vi "Parse file name.vi"(10 "filename without extension":string, 11 "File Path":path) -> (1 "Changed reg":u8, 2 "Part info":string[](array[string]), 3 "Part info Header":string[](array[string]))   [LabVIEW 2020]
uses:
  XML Handler/XML Handler.lvclass
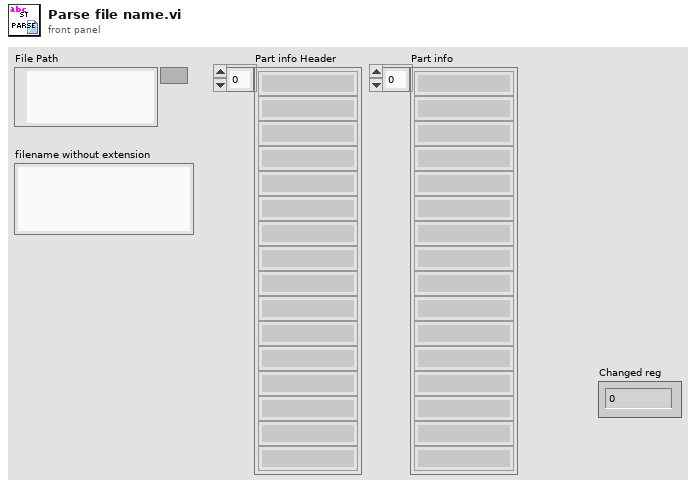
[diagram p1: front panel]
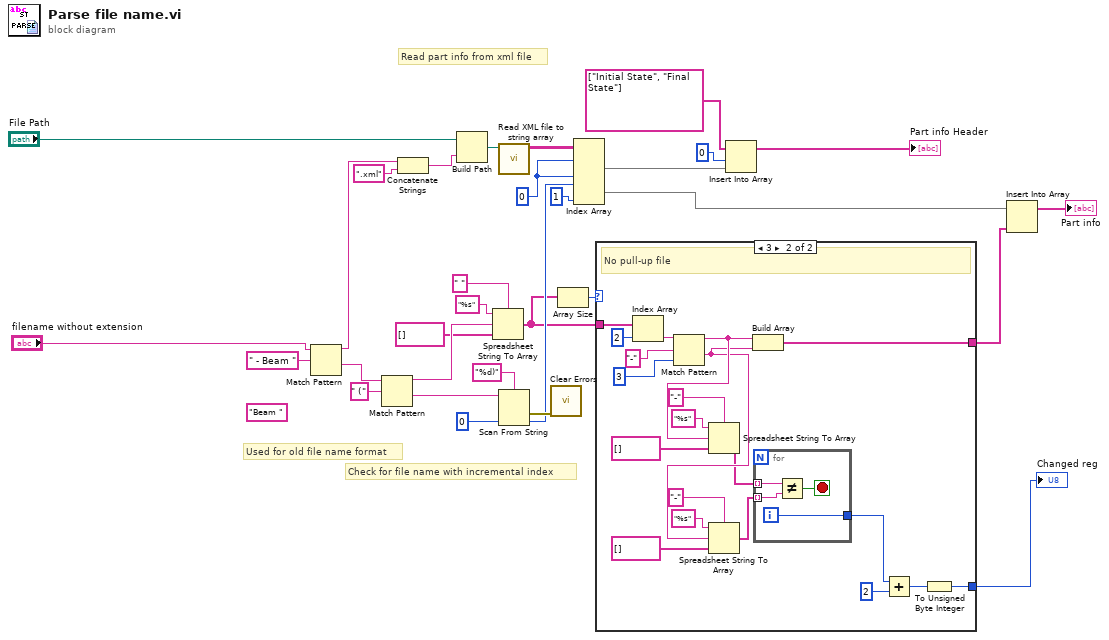
[diagram p0: block diagram]
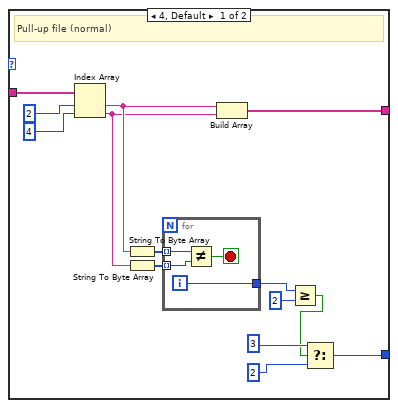
[diagram p2: hidden frame]
diagram:
  (unwired) "Beam " ("regular expression")
  w23 = 0 ("disabled index (page)")
  # "Used for old file name format"
  # "Check for file name with incremental index"
  # "Read part info from xml file"
  n1 = Match Pattern(string="filename without extension", regular expression=" - Beam ") -> (before substring=w25:string, after substring=w30:string)  [unwired: 1 in, 2 out]
  n2 = Match Pattern(string=w30, regular expression=" (") -> (before substring=w19:string, after substring=w18:string)  [unwired: 1 in, 2 out]
  n3 = Concatenate Strings(w25, ".xml" ("string")) -> (w24:string)
  n4 = Build Path(base path="File Path", name or relative path=w24) -> (appended path=w31:path)
  n5 = Spreadsheet String To Array(delimiter (Tab)=" ", format string="%s", spreadsheet string=w19, array type (2D Dbl)=string[] []) -> (array=w6:string[])
  n6 = call "Read XML file to string array.vi"("path to XML document"=w31) -> ("Array"=w11:string[][][])  [unwired: 9 in, 1 out]
  n7 = Scan From String(format string="%d)", input string=w18, default 1=0 ("default value 1")) -> (error out=w22:errorcluster, output 1=w21:i32)  [unwired: 2 in, 2 out]
  n8 = call <vilib>:"Clear Errors.vi"("error in (no error)"=w22) -> ()  [unwired: 5 in, 2 out]
  n9 = Array Size(array=w6) -> (size(s)=w5:i32)
  n10 = Index Array(array=w11, index (dim 0) #1=w23, index (dim 2) #1=w23, index (dim 0) #2=w21, index (dim 2) #2=1 ("disabled index (col)")) -> (element #1=w9:string[], element #2=w3:string[])  [unwired: 2 in]
  n11 = case shown="3" w5 {
    tunnel: w6 -> [w45 w69]
    tunnel: [w42 w64] -> w4
    tunnel: [w34 w50] -> w1
    frame 4, Default {
      # "Pull-up file (normal)"
      n12 = Index Array(array=w45, index #1=2 ("index"), index #2=4 ("index")) -> (element #1=w33:string, element #2=w32:string)
      n13 = String To Byte Array(string=w33) -> (unsigned byte array=w41:u8[])
      n14 = String To Byte Array(string=w32) -> (unsigned byte array=w40:u8[])
      n15 = for {
        tunnel: w41 -> [w49] mode=indexing
        tunnel: w40 -> [w48] mode=indexing
        tunnel: [w46] -> w39
        i -> [w46]
        stop <- w47 stop-if-true
        n16 = Not Equal?(x=w49, y=w48) -> (x != y?=w47:bool)
      }
      n17 = Build Array(w33, w32) -> (w42:string[])
      n18 = Greater Or Equal?(x=w39, y=2) -> (x >= y?=w35:bool)
      n19 = Select(t=u8 3, s=w35, f=u8 2) -> (s? t:f=w34:u8)
    }
    frame 3 {
      # "No pull-up file"
      n20 = Index Array(array=w69, index=2) -> (element=w67:string)
      n21 = Match Pattern(string=w67, regular expression="-", offset (0)=3) -> (before substring=w57:string, after substring=w56:string)  [unwired: 2 out]
      n22 = Spreadsheet String To Array(delimiter (Tab)="-", format string="%s", spreadsheet string=w57, array type (2D Dbl)=string[] []) -> (array=w54:string[])
      n23 = Spreadsheet String To Array(delimiter (Tab)="-", format string="%s", spreadsheet string=w56, array type (2D Dbl)=string[] []) -> (array=w55:string[])
      n24 = Build Array(w57, w56) -> (w64:string[])
      n25 = for {
        tunnel: w54 -> [w73] mode=indexing
        tunnel: w55 -> [w72] mode=indexing
        tunnel: [w70] -> w53
        i -> [w70]
        stop <- w71 stop-if-true
        n26 = Not Equal?(x=w73, y=w72) -> (x != y?=w71:bool)
      }
      n27 = Add(x=w53, y=2) -> (x+y=w51:i32)
      n28 = To Unsigned Byte Integer(number=w51) -> (unsigned 8bit integer=w50:u8)
    }
  }
  "Changed reg" <- w1
  n29 = Insert Into Array(array=string[] ["Initial State", "Final State"] ("Heading 2"), index=0, new element=w9) -> (→"Part info Header":string[])
  n30 = Insert Into Array(array=w3, new element=w4) -> (→"Part info":string[])  [unwired: 1 in]
